vi "Power meter.vi"(11 "VISA resource name":refnum<visa-resource-name>) -> (0 "error out":errorcluster)   [LabVIEW 2021, in "Ceyear.lvlib"]
uses:
  <instrlib>/Ceyear/Ceyear.lvlib
panel:
  out "Meas category":string
  in  "Exit":bool
  out "XY Graph":T1(graph)
  out "Power, mW":dbl(knob) scale=0.0..3.0
  out "VISA out":refnum<visa-resource-name>
  in  "L mean (nm)":dbl=955.0 format="%.2f"
  in  "Stop PM":bool
  in  "Start PM":bool
  in  "Apply":bool
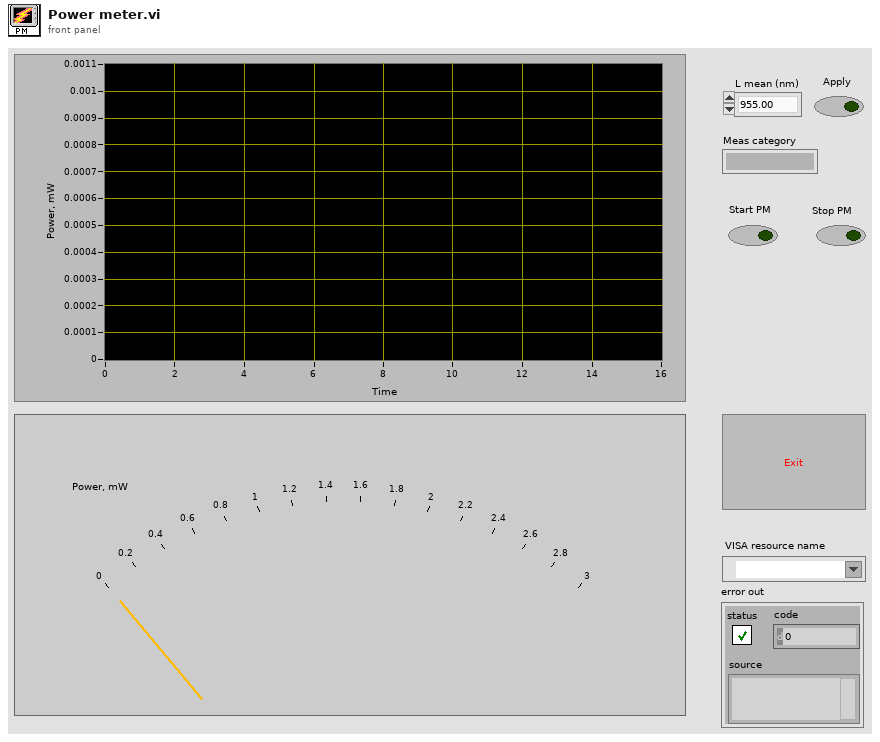
[diagram p1: front panel]
types:
  T1 = cluster{"array type (2D Dbl)":dbl[], "array type (2D Dbl)":dbl[]}
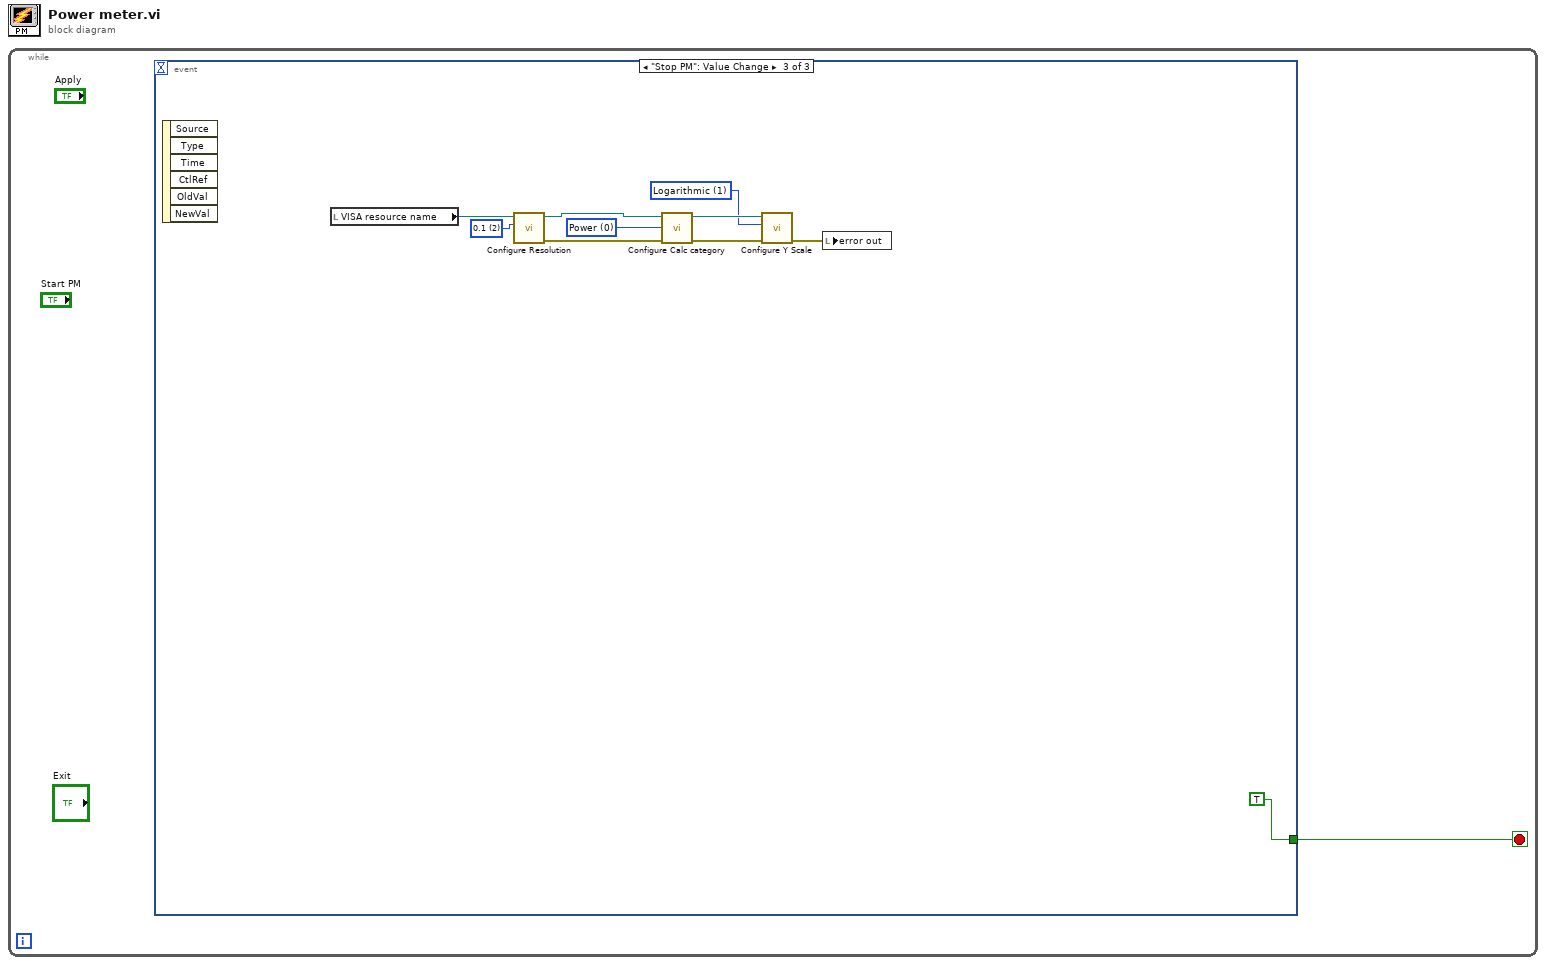
[diagram p0: block diagram]
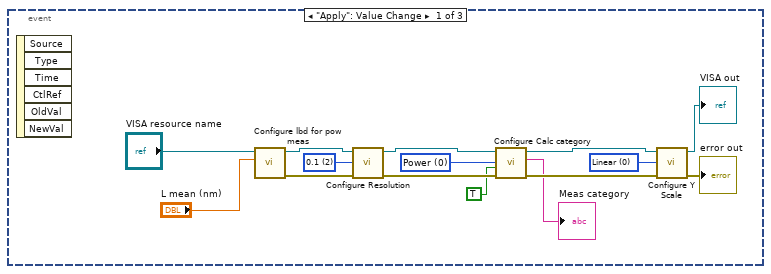
[diagram p2: hidden frame]
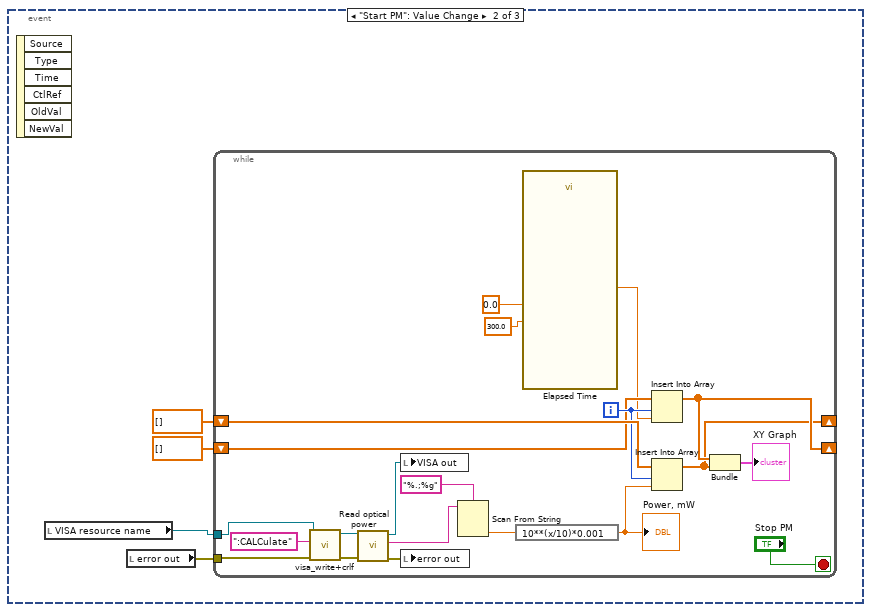
[diagram p3: hidden frame]
diagram:
  n1 = while {
    stop <- w1 stop-if-true
    n2 = event shown="[2] \"Stop PM\": Value Change" {
      selector: _ -> [_ _ _]
      dyn-events: _ -> [_ _ _]
      timeout: _ -> [_ _ _]
      tunnel: [_ _ TRUE] -> w1
      event "Apply": Value Change {
        w6 = u16 0 items=["Linear", "Logarithmic"] ("Spacing")
        w5 = u16 0 items=["Power", "SMSR"] ("Category")
        w4 = u16 2 items=["0.02", "0.05", "0.1", "0.2", "0.5", "1", "2"] ("Resolution (nm)")
        n3 = event-data() -> ()  [unwired: 1 in, 6 out]
        n4 = call <instrlib>:"Configure lbd for pow meas.vi"("Meas lbd (span 0.1 nm)"="L mean (nm)", "VISA resource name"="VISA resource name") -> ("error out"=w7:errorcluster, "VISA resource name out"=w8:refnum<visa-resource-name>)  [unwired: 8 in]
        n5 = call <instrlib>:"Configure Resolution.vi"("error in (no error)"=w7, "Resolution (nm)"=w4, "VISA resource name"=w8) -> ("error out"=w10:errorcluster, "VISA resource name out"=w9:refnum<visa-resource-name>)  [unwired: 7 in]
        n6 = call <instrlib>:"Configure Calc category.vi"("error in (no error)"=w10, "ask_ category"=TRUE, "Category"=w5, "VISA resource name"=w9) -> ("error out"=w12:errorcluster, "Category"=→"Meas category":string, "VISA resource name out"=w11:refnum<visa-resource-name>)  [unwired: 5 in]
        n7 = call <instrlib>:"Configure Y Scale.vi"("error in (no error)"=w12, "Spacing"=w6, "VISA resource name"=w11) -> ("error out"=→"error out":errorcluster, "VISA resource name out"=→"VISA out":refnum<visa-resource-name>)  [unwired: 7 in]
      }
      event "Start PM": Value Change {
        n8 = event-data() -> ()  [unwired: 1 in, 6 out]
        n9 = local read "VISA resource name"() -> (w18:refnum<visa-resource-name>)
        n10 = local read "error out"() -> (w17:errorcluster)
        n11 = while {
          shift-right: [w33] -> _
          shift-left: dbl[] [] ("array type (2D Dbl)") -> [w37]
          shift-right: [w34] -> _
          shift-left: dbl[] [] ("array type (2D Dbl)") -> [w35]
          tunnel: w18 -> [w24]
          tunnel: w17 -> [w23]
          i -> [w36]
          stop <- "Stop PM" stop-if-true
          n12 = call <instrlib>:"visa_write+crlf.vi"("error in (no error)"=w23, "Strings (empty)"=":CALCulate" ("write buffer"), "VISA resource name"=w24) -> ("error out"=w22:errorcluster, "VISA resource name out"=w21:refnum<visa-resource-name>)  [unwired: 7 in]
          n13 = call <instrlib>:"Read optical power.vi"("error in (no error)"=w22, "VISA resource name"=w21) -> ("error out"=w39:errorcluster, "data"=w29:string, "VISA resource name out"=w40:refnum<visa-resource-name>)  [unwired: 7 in]
          n14 = local write "VISA out"(w40) -> ()
          n15 = local write "error out"(w39) -> ()
          n16 = Scan From String(format string="%.;%g", input string=w29) -> (output 1=w31:dbl)  [unwired: 3 in, 3 out]
          n17 = expression code="10**(x/10)*0.001"(w31) -> (w30:dbl)
          "Power, mW" <- w30
          n18 = call "Elapsed Time"("Time Target (s)"=300.0, "Set Start Time (s)"=0.0) -> ("Elapsed Time (s)"=w27:dbl)  [unwired: 10 in, 7 out]
          n19 = Insert Into Array(array=w35, index=w36, new element=w27) -> (w34:dbl[])
          n20 = Insert Into Array(array=w37, index=w36, new element=w30) -> (w33:dbl[])
          n21 = Bundle("array type (2D Dbl)"=w34, "array type (2D Dbl)"=w33) -> (→"XY Graph":T1)  [unwired: 1 in]
        }
      }
      event "Stop PM": Value Change {
        w45 = u16 1 items=["Linear", "Logarithmic"] ("Spacing")
        w44 = u16 0 items=["Power", "SMSR"] ("Category")
        w43 = u16 2 items=["0.02", "0.05", "0.1", "0.2", "0.5", "1", "2"] ("Resolution (nm)")
        n22 = event-data() -> ()  [unwired: 1 in, 6 out]
        n23 = local read "VISA resource name"() -> (w50:refnum<visa-resource-name>)
        n24 = call <instrlib>:"Configure Resolution.vi"("Resolution (nm)"=w43, "VISA resource name"=w50) -> ("error out"=w47:errorcluster, "VISA resource name out"=w46:refnum<visa-resource-name>)  [unwired: 8 in]
        n25 = call <instrlib>:"Configure Calc category.vi"("error in (no error)"=w47, "Category"=w44, "VISA resource name"=w46) -> ("error out"=w49:errorcluster, "VISA resource name out"=w48:refnum<visa-resource-name>)  [unwired: 6 in, 1 out]
        n26 = call <instrlib>:"Configure Y Scale.vi"("error in (no error)"=w49, "Spacing"=w45, "VISA resource name"=w48) -> ("error out"=w51:errorcluster)  [unwired: 7 in, 1 out]
        n27 = local write "error out"(w51) -> ()
      }
    }
  }
